vi "Edit_First_Equal.vi"(1 "String in":string) -> (0 "String out":string)   [LabVIEW 2014]
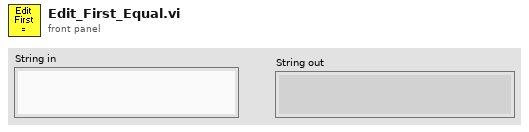
[diagram p1: front panel]
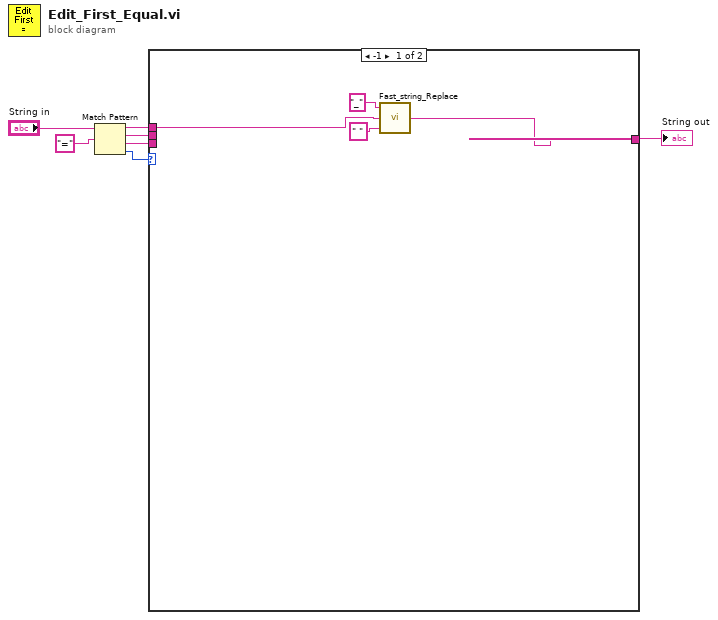
[diagram p0: block diagram]
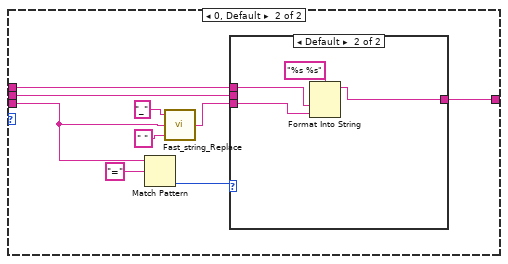
[diagram p2: hidden frame]
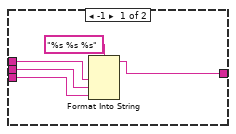
[diagram p3: hidden frame]
diagram:
  n1 = Match Pattern(string="String in", regular expression="=") -> (before substring=w3:string, match substring=w4:string, after substring=w5:string, offset past match=w7:i32)  [unwired: 1 in]
  n2 = case shown="-1" w7 {
    tunnel: w3 -> [w9 w20]
    tunnel: w4 -> [_ w19]
    tunnel: w5 -> [_ w13]
    tunnel: [w8 w18] -> w6
    frame -1 {
      n3 = call "Fast_string_Replace.vi"("Replace match with:"=" ", "Input String"=w9, "regular expression"="_") -> ("Output String"=w8:string)  [unwired: 2 out]
    }
    frame 0, Default {
      n4 = Match Pattern(string=w13, regular expression="=") -> (offset past match=w16:i32)  [unwired: 1 in, 3 out]
      n5 = call "Fast_string_Replace.vi"("Replace match with:"=" ", "Input String"=w13, "regular expression"="_") -> ("Output String"=w12:string)  [unwired: 2 out]
      n6 = case shown="Default" w16 {
        tunnel: w20 -> [w25 w29]
        tunnel: w19 -> [w24 _]
        tunnel: [w23 w28] -> w18
        tunnel: w12 -> [w21 w26]
        frame -1 {
          n7 = Format Into String(format string="%s %s %s", w25, w24, w21) -> (resulting string=w23:string)  [unwired: 2 in, 1 out]
        }
        frame Default {
          n8 = Format Into String(format string="%s %s", w29, w26) -> (resulting string=w28:string)  [unwired: 2 in, 1 out]
        }
      }
    }
  }
  "String out" <- w6
